vi "Cut Length.vi"(5 "y2":dbl, 7 "y1":dbl, 9 "x2":dbl, 10 "x1":dbl, 11 "circle":cluster{"x0":dbl, "y0":dbl, "r":dbl}) -> (3 "length":dbl)   [LabVIEW 2023]
doc: "Calculates the cut length."
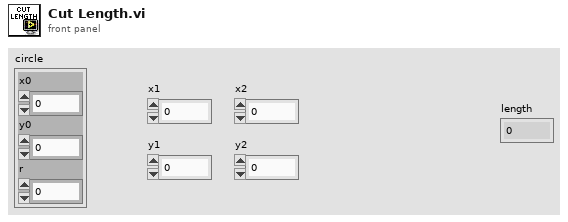
[diagram p1: front panel]
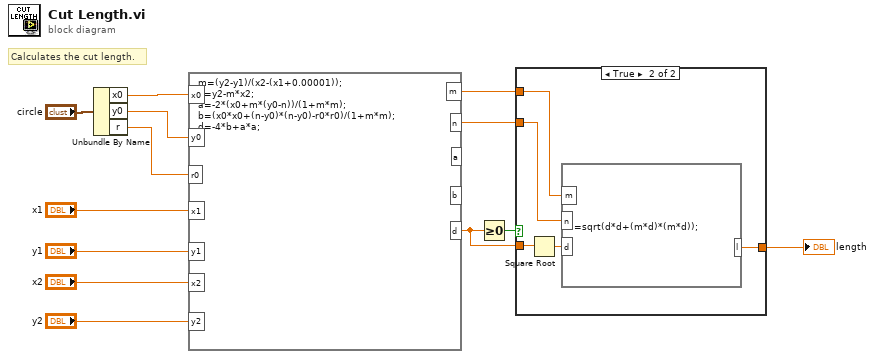
[diagram p0: block diagram]
diagram:
  # "Calculates the cut length."
  n1 = Unbundle By Name("circle") -> ("x0"=w3:dbl, "y0"=w2:dbl, "r"=w1:dbl)
  n2 = formula code="m=(y2-y1)/(x2-(x1+0.00001));\nn=y2-m*x2;\na=-2*(x0+m*(y0-n))/(1+m*m);\nb=(x0*x0+(n-y0)*(n-y0)-r0*r0)/(1+m*m);\nd=-4*b+a*a;"("x0"=w3, "y0"=w2, "r0"=w1, "x1"="x1", "y1"="y1", "x2"="x2", "y2"="y2") -> ("m"=w7:dbl, "n"=w6:dbl, "d"=w5:dbl)  [unwired: 2 out]
  n3 = Greater Or Equal To 0?(x=w5) -> (x >= 0?=w9:bool)
  n4 = case shown="True" w9 {
    tunnel: w5 -> [_ w18]
    tunnel: [_ w14] -> w8
    tunnel: w7 -> [_ w17]
    tunnel: w6 -> [_ w16]
    frame False {
    }
    frame True {
      n5 = Square Root(x=w18) -> (sqrt(x)=w15:dbl)
      n6 = formula code="l=sqrt(d*d+(m*d)*(m*d));"("m"=w17, "n"=w16, "d"=w15) -> ("l"=w14:dbl)
    }
  }
  "length" <- w8
